vi "Configure PRACH Limit Phase Error.vi"(5 "Peak (0.0)":dbl format="%^.3e", 6 "Peak Enabled (Off)":i32(ring) items=["Off", "On", "Value"], 7 "RMS (0.0)":dbl format="%^.3e", 8 "error in (no error)":errorcluster, 9 "RMS Enabled (Off)":i32(ring) items=["Off", "On", "Value"], 10 "Instance (1)":T1=1, 11 "VISA resource name":refnum<visa-resource-name>) -> (0 "error out":errorcluster, 3 "VISA resource name out":refnum<visa-resource-name>)   [LabVIEW 2020, in "Rohde&Schwarz CMWXP NR FR1 Measurement.lvlib"]
doc: "Defines symmetric limits for the RMS and peak values of the phase error. The limit check fails if the absolute value of the measured phase error exceeds the specified values.\n\nAttribute:\nRSCMWXPNRFR1M_ATTR_PRACH_LIMIT_PHASE_ERROR\n\nRemote-control command:\nCONFigure:NRSub:MEAS<i>:PRACh:LIMit:PERRor"
uses:
  <instrlib>/Rohde&Schwarz CMWXP NR FR1 Measurement/Rohde&Schwarz CMWXP NR FR1 Measurement.lvlib
  <instrlib>/Rohde&Schwarz CMWXP NR FR1 Measurement/Private/_Instance.ctl
  <instrlib>/Rohde&Schwarz CMWXP NR FR1 Measurement/Private/rsidr_core.llb/rsidr_core.lvlib
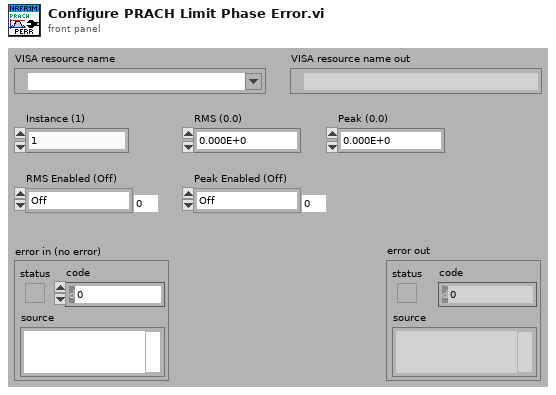
[diagram p1: front panel]
types:
  T1 = typedef "Rohde&Schwarz CMWXP NR FR1 Measurement.lvlib/_Instance.ctl" = i32
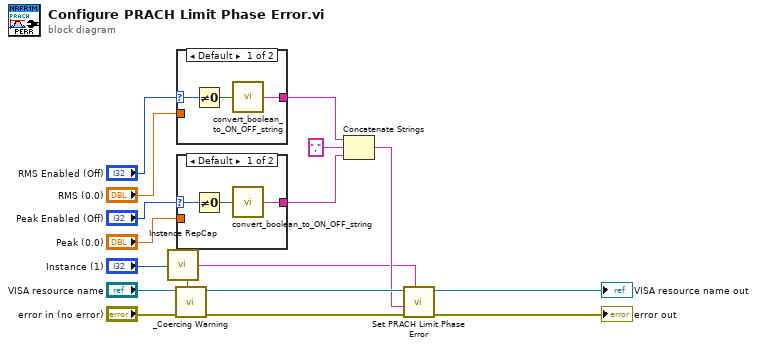
[diagram p0: block diagram]
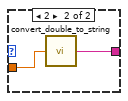
[diagram p2: hidden frame]
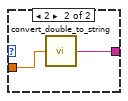
[diagram p3: hidden frame]
diagram:
  n1 = call <instrlib>:"Instance RepCap.vi"("Instance In"="Instance (1)") -> ("In Range?"=w12:bool, "RepCap Identifier Out"=w2:string)  [unwired: 1 in]
  n2 = call <instrlib>:"_Coercing Warning.vi"("In Range?"=w12, "error in (no error)"="error in (no error)", "VISA resource name"="VISA resource name") -> ("error out"=w15:errorcluster, "VISA resource name out"=w14:refnum<visa-resource-name>)  [unwired: 7 in]
  n3 = case shown="Default" "RMS Enabled (Off)" {
    selector: "RMS Enabled (Off)" -> [w20 _]
    tunnel: "RMS (0.0)" -> [_ w22]
    tunnel: [w18 w21] -> w5
    frame Default {
      n4 = Not Equal To 0?(x=w20) -> (x != 0?=w19:bool)
      n5 = call <instrlib>:"convert_boolean_to_ON_OFF_string.vi"("boolean value in"=w19) -> ("string value out"=w18:string)  [unwired: 4 in]
    }
    frame 2 {
      n6 = call <instrlib>:"convert_double_to_string.vi"("double in"=w22) -> ("string out"=w21:string)  [unwired: 4 in]
    }
  }
  n7 = case shown="Default" "Peak Enabled (Off)" {
    selector: "Peak Enabled (Off)" -> [w25 _]
    tunnel: "Peak (0.0)" -> [_ w27]
    tunnel: [w23 w26] -> w4
    frame Default {
      n8 = Not Equal To 0?(x=w25) -> (x != 0?=w24:bool)
      n9 = call <instrlib>:"convert_boolean_to_ON_OFF_string.vi"("boolean value in"=w24) -> ("string value out"=w23:string)  [unwired: 4 in]
    }
    frame 2 {
      n10 = call <instrlib>:"convert_double_to_string.vi"("double in"=w27) -> ("string out"=w26:string)  [unwired: 4 in]
    }
  }
  n11 = Concatenate Strings(w5, ",", w4) -> (w3:string)
  n12 = call "Set PRACH Limit Phase Error"("Repeated Capabilities"=w2, "error in (no error)"=w15, "PRACH Limit Phase Error ()"=w3, "instrument handle"=w14) -> ("error out"=→"error out":errorcluster, "instrument handle out"=→"VISA resource name out":refnum<visa-resource-name>)  [unwired: 6 in]
